vi "WSVCAP SHL Host LL I2C Build Socket Mask.vi"(0 "DUT Mask Array":bool[][](array[boolean]), 7 "DUT Mask Mode (Custom)":T1) -> (4 "Socket Mask [U64]":u64 format="%012x", 8 "Socket Mask Array":bool[][](array[boolean]))   [LabVIEW 2012]
uses:
  Type Defs/WSVCAP SHL DUT Number Enum.ctl
  Type Defs/WSVCAP SHL I2C DUT Mask Mode Enum.ctl
panel:
  in  "DUT":T2
  # "DUT 01"
  # "DUT 02"
  # "DUT 03"
  # "DUT 04"
  # "DUT 05"
  # "DUT 06"
  # "DUT 07"
  # "DUT 08"
  # "DUT 09"
  # "DUT 10"
  # "DUT 11"
  # "DUT 12"
  # "DUT 13"
  # "DUT 14"
  # "DUT 15"
  # "DUT 16"
  # "C1"
  # "C2"
  # "C3"
  # "SKT 01"
  # "SKT 02"
  # "SKT 03"
  # "SKT 04"
  # "SKT 05"
  # "SKT 06"
  # "SKT 07"
  # "SKT 08"
  # "SKT 09"
  # "SKT 10"
  # "SKT 11"
  # "SKT 12"
  # "SKT 13"
  # "SKT 14"
  # "SKT 15"
  # "SKT 16"
  # "C1"
  # "C2"
  # "C3"
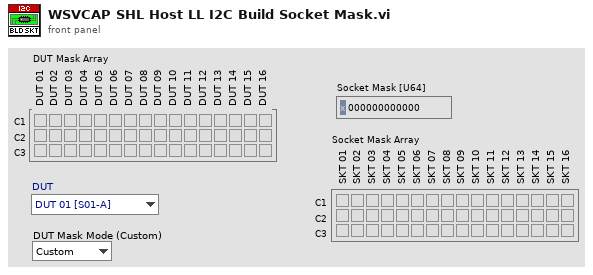
[diagram p1: front panel]
types:
  T1 = typedef "WSVCAP SHL I2C DUT Mask Mode Enum.ctl" = enum16{"Custom", "C1", "C2", "C3", "All"}
  T2 = typedef "WSVCAP SHL DUT Number Enum.ctl" = enum16{"DUT 01 [S01-A]", "DUT 02 [S02-B]", "DUT 03 [S03-C]", "DUT 04 [S04-D]", "DUT 05 [S05-E]", "DUT 06 [S06-F]", "DUT 07 [S07-G]", "DUT 08 [S08-H]", "DUT 09 [S09-I]", "DUT 10 [S10-J]", "DUT 11 [S11-K]", "DUT 12 [S12-L]", "DUT 13 [S13-M]", "DUT 14 [S14-N]", "DUT 15 [S15-O]", "DUT 16 [S16-P]"}
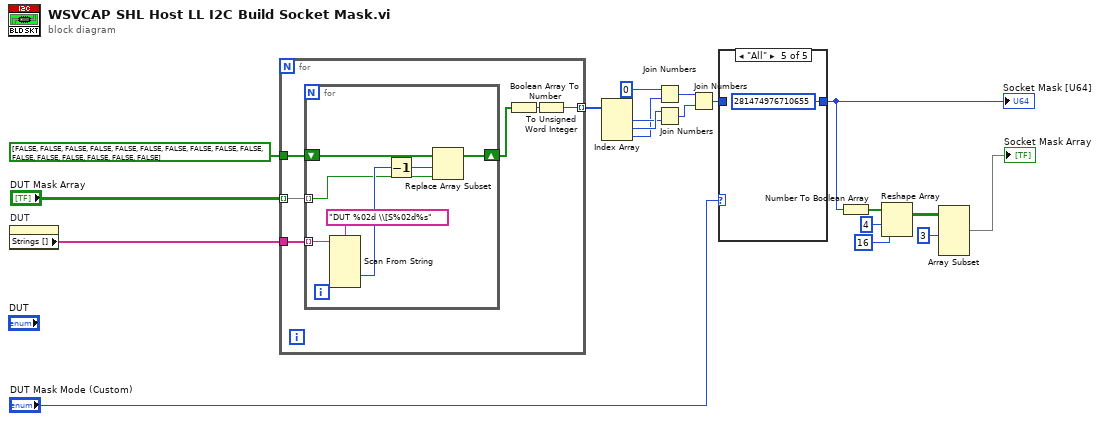
[diagram p0: block diagram]
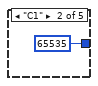
[diagram p3: hidden frame]
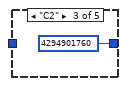
[diagram p4: hidden frame]
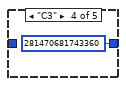
[diagram p5: hidden frame]
diagram:
  n1 = property on="DUT" class="Enum (strict)"() -> ("Strings []"=w18:string[])  [unwired: 2 in, 2 out]
  n2 = for {
    tunnel: bool[] [FALSE, FALSE, FALSE, FALSE, FALSE, FALSE, FALSE, FALSE, FALSE, FALSE, FALSE, FALSE, FALSE, FALSE, FALSE, FALSE] -> [w25]
    tunnel: w18 -> [w24]
    tunnel: "DUT Mask Array" -> [w23] mode=indexing
    tunnel: [w20] -> w16 mode=indexing
    n3 = for {
      tunnel: w24 -> [w32] mode=indexing
      tunnel: w23 -> [w27] mode=indexing
      shift-right: [w29] -> w21
      shift-left: w25 -> [w30]
      n4 = Scan From String(format string="DUT %02d \\[S%02d%s", input string=w32) -> (output 2=w28:i32)  [unwired: 7 in, 3 out]
      n5 = Decrement(x=w28) -> (x-1=w26:i32)
      n6 = Replace Array Subset(array=w30, new element=w27, index=w26) -> (w29:bool[])
    }
    n7 = Boolean Array To Number(Boolean array=w21) -> (number=w22:u32)
    n8 = To Unsigned Word Integer(number=w22) -> (unsigned 16bit integer=w20:u16)
  }
  n9 = Index Array(array=w16) -> (element #1=w14:u16, element #2=w15:u16, element #3=w13:u16)  [unwired: 3 in]
  n10 = Join Numbers(hi=u16 0, lo=w13) -> ((hi.lo)=w11:u32)
  n11 = Join Numbers(hi=w15, lo=w14) -> ((hi.lo)=w10:u32)
  n12 = Join Numbers(hi=w11, lo=w10) -> ((hi.lo)=w8:u64)
  n13 = case shown="\"All\"" "DUT Mask Mode (Custom)" {
    tunnel: [w33 u64 65535 ("Socket Mask [U64]") u64 4294901760 ("Socket Mask [U64]") u64 281470681743360 ("Socket Mask [U64]") u64 281474976710655 ("Socket Mask [U64]")] -> w7
    tunnel: w8 -> [w33 _ _ _ _]
    frame "Custom" {
    }
    frame "C1" {
    }
    frame "C2" {
    }
    frame "C3" {
    }
    frame "All" {
    }
  }
  "Socket Mask [U64]" <- w7
  n14 = Number To Boolean Array(number=w7) -> (Boolean array=w6:bool[])
  n15 = Reshape Array(w6, 4 ("dimension size"), 16 ("dimension size")) -> (w3:bool[][])
  n16 = Array Subset(array=w3, length (row)=3 ("length")) -> (→"Socket Mask Array":bool[][])  [unwired: 3 in]
